vi "Get_Trck_Group_Frames_Visual-3.vi"(5 "Dot Status IN":i16[][](array[numeric]), 6 "error IN":errorcluster, 7 "Start Pos IN":i32[](array[numeric]), 8 "Track ID IN":u16[](array[numeric]), 9 "Tracks IN":dbl[][](array[numeric])) -> (0 "error OUT":errorcluster, 3 "[OUT] Grou\nped Tracks":T1(array[cluster]))   [LabVIEW 2013]
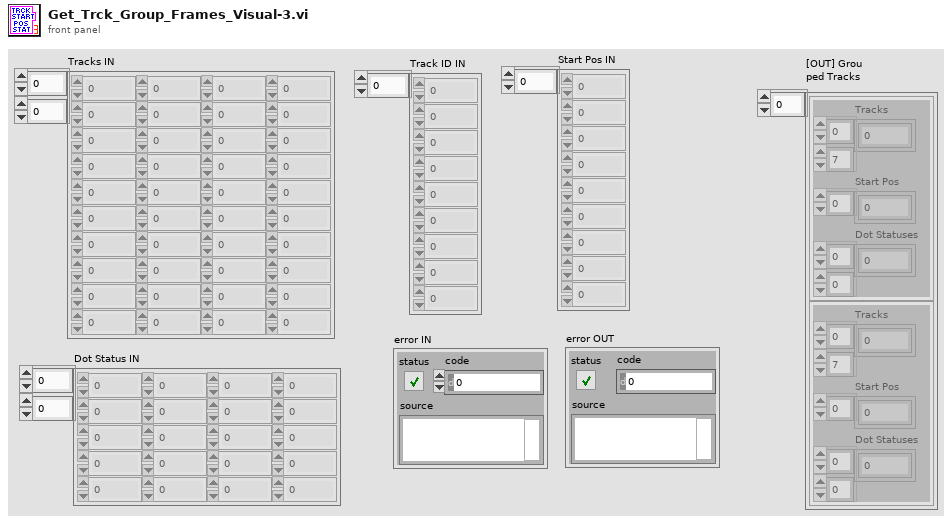
[diagram p1: front panel]
types:
  T1 = cluster{"Tracks":dbl[][], "Start Pos":i32[], "Dot Statuses":i16[][]}[]
  T2 = cluster{"Tracks":dbl[][], "Start Pos":i32[], "Dot Statuses":i16[][]}
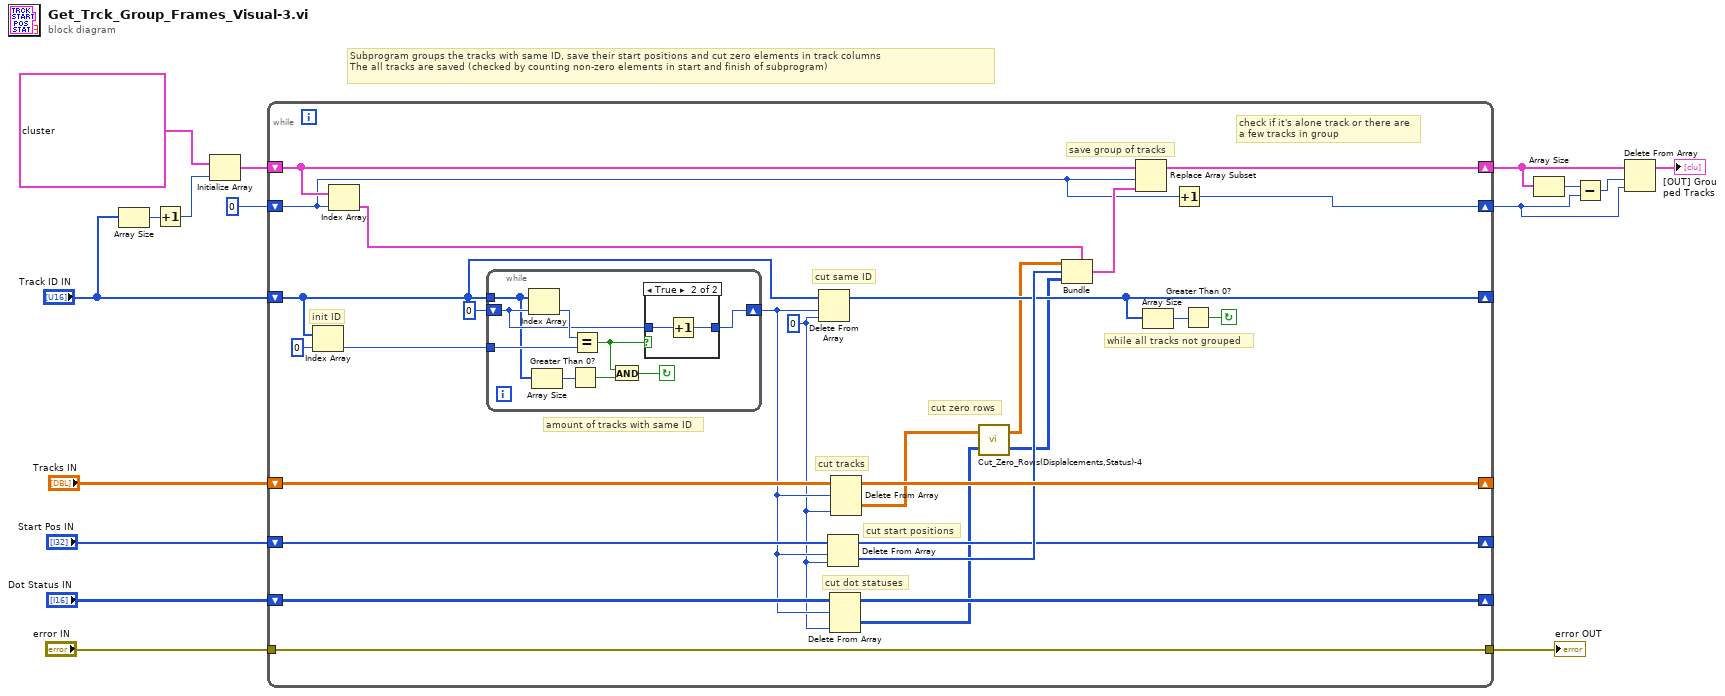
[diagram p0: block diagram]
diagram:
  # "Subprogram groups the tracks with same ID, save their start positions and cut zero elements in track columns \nThe all tracks are saved (checked by counting non-zero elements in start and finish of subprogram)"
  n1 = Array Size(array="Track ID IN") -> (size(s)=w12:i32)
  n2 = Increment(x=w12) -> (x+1=w16:i32)
  n3 = Initialize Array(T2 {"Tracks"=[], "Start Pos"=array[1605 elements], "Dot Statuses"=[]}, w16) -> (w5:T1)
  n4 = while {
    shift-right: [w27] -> w4
    shift-left: w5 -> [w31]
    shift-right: [w38] -> _
    shift-left: "Tracks IN" -> [w39]
    shift-right: [w34] -> _
    shift-left: "Track ID IN" -> [w41]
    shift-right: [w35] -> _
    shift-left: "Start Pos IN" -> [w37]
    shift-right: [w28] -> w6
    shift-left: 0 -> [w29]
    tunnel: "error IN" -> [w26]
    tunnel: [w26] -> w10
    shift-right: [w21] -> _
    shift-left: "Dot Status IN" -> [w24]
    stop <- w32 continue-if-true
    w22 = 0 ("index")
    # "save group of tracks"
    # "cut zero rows"
    # "cut dot statuses"
    # "check if it's alone track or there are\na few tracks in group"
    # "cut start positions"
    # "while all tracks not grouped"
    # "cut tracks"
    # "cut same ID"
    # "amount of tracks with same ID"
    # "init ID"
    n5 = Index Array(array=w41, index=0) -> (element=w25:u16)
    n6 = Index Array(array=w31, index=w29) -> (element=w40:T2)
    n7 = while {
      tunnel: w25 -> [w51]
      tunnel: w41 -> [w48]
      shift-right: [w49] -> w23
      shift-left: 0 -> [w50]
      stop <- w44 continue-if-true
      n8 = Index Array(array=w48, index=w50) -> (element=w52:u16)
      n9 = Array Size(array=w48) -> (size(s)=w47:i32)
      n10 = Greater Than 0?(x=w47) -> (x > 0?=w45:bool)
      n11 = Equal?(x=w52, y=w51) -> (x = y?=w46:bool)
      n12 = And(x=w46, y=w45) -> (x .and. y?=w44:bool)
      n13 = case shown="True" w46 {
        tunnel: w50 -> [w53 w55]
        tunnel: [w53 w54] -> w49
        frame False {
        }
        frame True {
          n14 = Increment(x=w55) -> (x+1=w54:i32)
        }
      }
    }
    n15 = Delete From Array(array=w41, length=w23, index=w22) -> (array with subset deleted=w34:u16[])  [unwired: 1 out]
    n16 = Delete From Array(array=w37, length=w23, index=w22) -> (deleted portion=w36:i32[], array with subset deleted=w35:i32[])
    n17 = Delete From Array(array=w24, length=w23, index (col)=w22) -> (deleted portion=w18:i16[][], array with subset deleted=w21:i16[][])  [unwired: 1 in]
    n18 = Delete From Array(array=w39, length=w23, index (col)=w22) -> (deleted portion=w20:dbl[][], array with subset deleted=w38:dbl[][])  [unwired: 1 in]
    n19 = call "Cut_Zero_Rows(Displalcements,Status)-4.vi"("[IN] Dot matrix\nwith zero points"=w18, "[IN] (X,Y,dX,dY) \nwith zero displ"=w20) -> ("[OUT] Dot \nMatrix"=w17:i16[][], "[OUT] (X,Y,dX,dY)\nw/t zero displac"=w19:dbl[][])
    n20 = Bundle(cluster=w40, "Tracks"=w19, "Start Pos"=w36, "Dot Statuses"=w17) -> (w30:T2)
    n21 = Replace Array Subset(array=w31, new element=w30, index=w29) -> (w27:T1)
    n22 = Array Size(array=w34) -> (size(s)=w33:i32)
    n23 = Increment(x=w29) -> (x+1=w28:i32)
    n24 = Greater Than 0?(x=w33) -> (x > 0?=w32:bool)
  }
  "error OUT" <- w10
  n25 = Array Size(array=w4) -> (size(s)=w9:i32)
  n26 = Subtract(x=w9, y=w6) -> (x-y=w8:i32)
  n27 = Delete From Array(array=w4, length=w8, index=w6) -> (array with subset deleted=→"[OUT] Grou\nped Tracks":T1)  [unwired: 1 out]
